vi "4155C QSCV v3.0.vi"(0 "VISA resource name in":refnum<visa-resource-name>="GPIB0::14::INSTR", 1 "Timings":T2={"hold time (sec)"=0.0, "delay time (sec)"=0.0, "Step Time (0 disables)"=0.0, "C-Step"=0.1, "CInt"=0.1, "IInt"=0.1} {"IInt" min=0.01 max=10.0 format="%.2f"; "CInt" min=0.01 max=10.0 format="%.2f"; "C-Step" min=0.01 max=10.0 format="%.2f"; "Step Time (0 disables)" min=0.0 format="%.2f"; "delay time (sec)" min=0.0 format="%.4f"; "hold time (sec)" min=0.0 format="%.4f"}, 2 "Drain":T4={"Drain voltage"=0.0, "Drain Compliance"=0.0001, "Range mode"=0, "Range"=6} {"Range" max=11 scale=0.0..11.0; "Range mode" items=["Auto", "Limited", "Fixed"]; "Drain Compliance" min=0.0 max=0.1 format="%^.2e"; "Drain voltage" min=-100.0 max=100.0 format="%^.4e"}, 3 "Gate":T3={"Gate Start"=0.0, "Gate Stop"=2.0, "Gate Step"=1.0, "Gate Compliance"=0.0001, "Range mode"=0, "Range"=6} {"Range" max=11 scale=0.0..11.0; "Range mode" items=["Auto", "Limited", "Fixed"]; "Gate Compliance" min=0.0 max=0.1 format="%^.2e"; "Gate Step" min=-100.0 max=100.0 format="%^.4e"; "Gate Stop" min=-100.0 max=100.0 format="%^.4e"; "Gate Start" min=-100.0 max=100.0 format="%^.4e"}, 4 "Panel Controls":T1={"Emergency Stop"=refnum, "CapGraph Max"=1e-05, "Text/Graph (text=false)"=FALSE} {"CapGraph Max" format="%.2e"}, 5 "error in (no error)":errorcluster, 6 "sweep mode":u16(ring) items=["Single", "Double"], 8 "QSCV - Source/Common":u32(ring) items=["SMU1  ", "SMU2  ", "SMU3  ", "SMU4  ", "SMU5  ", "SMU6  ", "VSU1  ", "VSU2  "], 9 "QSCV - Gate":u32(ring)=2 items=["SMU1  ", "SMU2  ", "SMU3  ", "SMU4  ", "SMU5  ", "SMU6  ", "VSU1  ", "VSU2  "], 10 "QSCV - Drain":u32(ring)=1 items=["SMU1  ", "SMU2  ", "SMU3  ", "SMU4  ", "SMU5  ", "SMU6  ", "VSU1  ", "VSU2  "], 11 "QSCV - Probe 4":u32(ring)=3 items=["SMU1  ", "SMU2  ", "SMU3  ", "SMU4  ", "SMU5  ", "SMU6  ", "VSU1  ", "VSU2  "]) -> (14 "VISA Resource Name out":refnum<visa-resource-name>, 15 "VG":dbl[](array[numeric]) format="%.2f", 16 "Cap":dbl[](array[numeric]) format="%.2f", 17 "Leak":dbl[](array[numeric]) format="%.2f", 18 "Number of points":i32=1, 19 "error out":errorcluster)   [LabVIEW 2016]
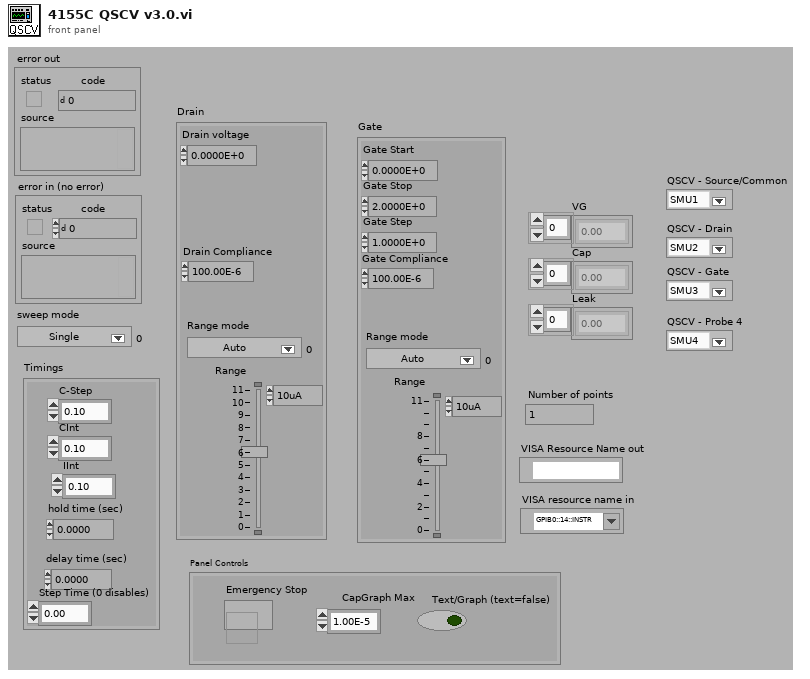
[diagram p1: front panel]
types:
  T1 = cluster{"Emergency Stop":refnum<vi>, "CapGraph Max":dbl, "Text/Graph (text=false)":bool}
  T2 = cluster{"hold time (sec)":dbl, "delay time (sec)":dbl, "Step Time (0 disables)":dbl, "C-Step":dbl, "CInt":dbl, "IInt":dbl}
  T3 = cluster{"Gate Start":dbl, "Gate Stop":dbl, "Gate Step":dbl, "Gate Compliance":dbl, "Range mode":u16, "Range":u8}
  T4 = cluster{"Drain voltage":dbl, "Drain Compliance":dbl, "Range mode":u16, "Range":u8}
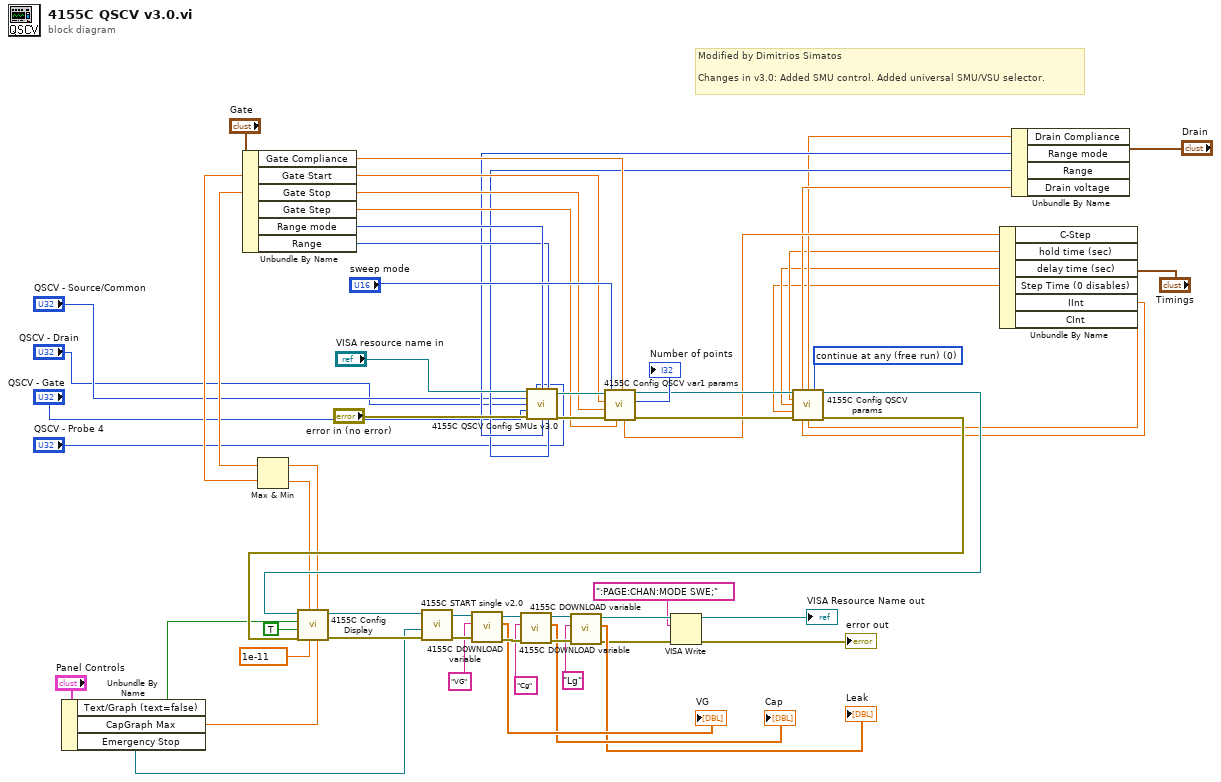
[diagram p0: block diagram]
diagram:
  w10 = u8 0 items=["continue at any (free run)", "stop at any abnorm", "stop at compliance"] ("stop condition (free run:0)")
  # "Modified by Dimitrios Simatos\n\nChanges in v3.0: Added SMU control. Added universal SMU/VSU selector."
  n1 = Unbundle By Name("Panel Controls") -> ("Text/Graph (text=false)"=w27:bool, "CapGraph Max"=w11:dbl, "Emergency Stop"=w29:refnum<vi>)
  n2 = Unbundle By Name("Gate") -> ("Gate Compliance"=w45:dbl, "Gate Start"=w33:dbl, "Gate Stop"=w32:dbl, "Gate Step"=w44:dbl, "Range mode"=w26:u16, "Range"=w25:u8)
  n3 = Max & Min(x=w32, y=w33) -> (max(x,y)=w30:dbl, min(x,y)=w31:dbl)
  n4 = Unbundle By Name("Timings") -> ("C-Step"=w19:dbl, "hold time (sec)"=w16:dbl, "delay time (sec)"=w15:dbl, "Step Time (0 disables)"=w14:dbl, "IInt"=w13:dbl, "CInt"=w12:dbl)
  n5 = Unbundle By Name("Drain") -> ("Drain Compliance"=w17:dbl, "Range mode"=w24:u16, "Range"=w23:u8, "Drain voltage"=w18:dbl)
  n6 = call "4155C QSCV Config SMUs v3.0.vi"("VISA resource name in"="VISA resource name in", "QSCV - Probe 4"="QSCV - Probe 4", "Gate mode"=w26, "Gate Range"=w25, "QSCV - Source/Common"="QSCV - Source/Common", "QSCV - Drain"="QSCV - Drain", "QSCV - Gate"="QSCV - Gate", "error in (no error)"="error in (no error)", "Source/drain mode"=w24, "Source/drain Range"=w23) -> ("VISA Resource Name out"=w51:refnum<visa-resource-name>, "error out"=w50:errorcluster)  [unwired: 4 in]
  n7 = call "4155C Config QSCV var1 params.vi"("Cap Step"=w19, "compliance"=w45, "step"=w44, "sweep mode"="sweep mode", "error in (no error)"=w50, "stop"=w32, "start"=w33, "VISA session"=w51) -> ("error out"=w20:errorcluster, "Number of points"=→"Number of points":i32, "dup VISA resource name"=w21:refnum<visa-resource-name>)  [unwired: 1 in]
  n8 = call "4155C Config QSCV params.vi"("VISA session"=w21, "Drain Voltage"=w18, "Drain Compliance"=w17, "stop condition (free run:0)"=w10, "HTIMe"=w16, "DELay"=w15, "RANGe"=w14, "error in (no error)"=w20, "I-Int"=w13, "C-Int"=w12) -> ("dup VISA resource name"=w34:refnum<visa-resource-name>, "error out"=w35:errorcluster)  [unwired: 4 in]
  n9 = call "4155C Config Display.vi"("Ymax"=w11, "Var1 Stop"=w30, "Ymin"=1e-11, "Var1 Start"=w31, "error in (no error)"=w35, "Logarithmic"=TRUE, "SPA Display"=w27, "VISA session"=w34) -> ("error out"=w36:errorcluster, "dup VISA resource name"=w37:refnum<visa-resource-name>)  [unwired: 2 in]
  n10 = call "4155C START single v2.0.vi"("error in (no error)"=w36, "Emergency Stop"=w29, "VISA resource name in"=w37) -> ("error out"=w60:errorcluster, "VISA Resource Name out"=w61:refnum<visa-resource-name>)  [unwired: 3 in]
  n11 = call "4155C DOWNLOAD variable.vi"("error in (no error)"=w60, "Variable name"="VG", "VISA resource name in"=w61) -> ("error out"=w58:errorcluster, "Output data"=→"VG":dbl[], "VISA Resource Name out"=w57:refnum<visa-resource-name>)  [unwired: 2 in]
  n12 = call "4155C DOWNLOAD variable.vi"("error in (no error)"=w58, "Variable name"="Cg", "VISA resource name in"=w57) -> ("error out"=w54:errorcluster, "Output data"=→"Cap":dbl[], "VISA Resource Name out"=w55:refnum<visa-resource-name>)  [unwired: 2 in]
  n13 = call "4155C DOWNLOAD variable.vi"("error in (no error)"=w54, "Variable name"="Lg", "VISA resource name in"=w55) -> ("error out"=w6:errorcluster, "Output data"=→"Leak":dbl[], "VISA Resource Name out"=w9:refnum<visa-resource-name>)  [unwired: 2 in]
  n14 = VISA Write(VISA resource name=w9, write buffer=":PAGE:CHAN:MODE SWE;" ("write buffer (\"\")"), error in (no error)=w6) -> (VISA resource name out=→"VISA Resource Name out":refnum<visa-resource-name>, error out=→"error out":errorcluster)  [unwired: 1 out]
